vi "Get Class Name.vi"(4 "LabVIEW Object":refnum<class>) -> (0 "Simple Name without Extension":string, 1 "Simple Name with Extension":string, 2 "Qualified Name":string)   [LabVIEW 2020, in "Utilities.lvlib"]
doc: "Gets the LabVIEW object's class name in various formats.\n\nAn example of the formats:\nQualified Name: Actor Extension.lvlib:Actor Extension.lvclass\nSimple Name with Extension: Actor Extension.lvclass\nSimple Name without Extension: Actor Extension"
uses:
  Utilities.lvlib
  <vilib>/regexp/Match Regular Expression.xnode
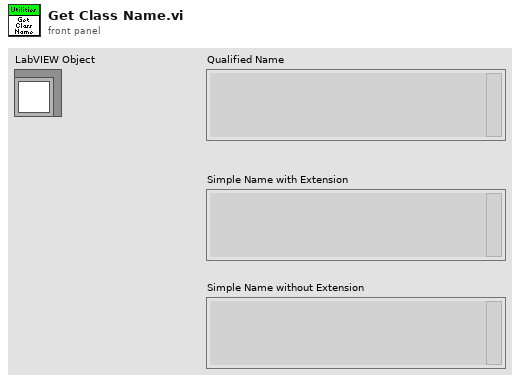
[diagram p1: front panel]
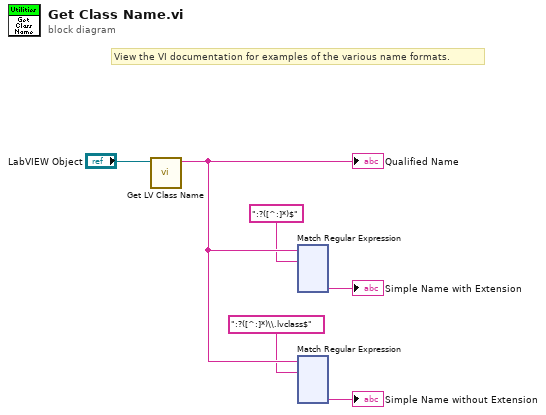
[diagram p0: block diagram]
diagram:
  # "View the VI documentation for examples of the various name formats."
  n1 = call <vilib>:"Get LV Class Name.vi"("object"="LabVIEW Object") -> ("class name"=w4:string)  [unwired: 9 in, 1 out]
  "Qualified Name" <- w4
  n2 = xnode "Match Regular Expression"("input string"=w4, "regular expression"=":?([^:]*)$") -> ("submatch 1"=→"Simple Name with Extension":string)  [unwired: 4 in, 5 out]
  n3 = xnode "Match Regular Expression"("input string"=w4, "regular expression"=":?([^:]*)\\.lvclass$") -> ("submatch 1"=→"Simple Name without Extension":string)  [unwired: 4 in, 5 out]
